vi "Source-meter - IV sweep.vi"(4 "XY Graph to update":refnum<vi>, 6 "String reference":refnum<vi>, 8 "Error In":errorcluster, 9 "Stop occurrence":refnum<k4>, 10 "IV properties":T1={"T"=0.0, "Vstart"=-0.5, "Vstop"=0.5, "Vpoints"=10.0, "Settling"=0.01, "I limit"=0.1, "Log mapping"=FALSE, "Averaging"=0.0}, 11 "Source-meter handle":T2) -> (0 "error out":errorcluster, 2 "Voltage (V)":dbl[](array[numeric]), 3 "Current (A)":dbl[](array[numeric]))   [LabVIEW 2019]
doc: "Handles I-V sweep (including data acquisition)"
uses:
  Type defs/Source-meter handle Type Def.ctl
  Type defs/Source-meter Type Def.ctl
  Custom devices/Custom source-meter settings.ctl
  Type defs/IV properties Type Def.ctl
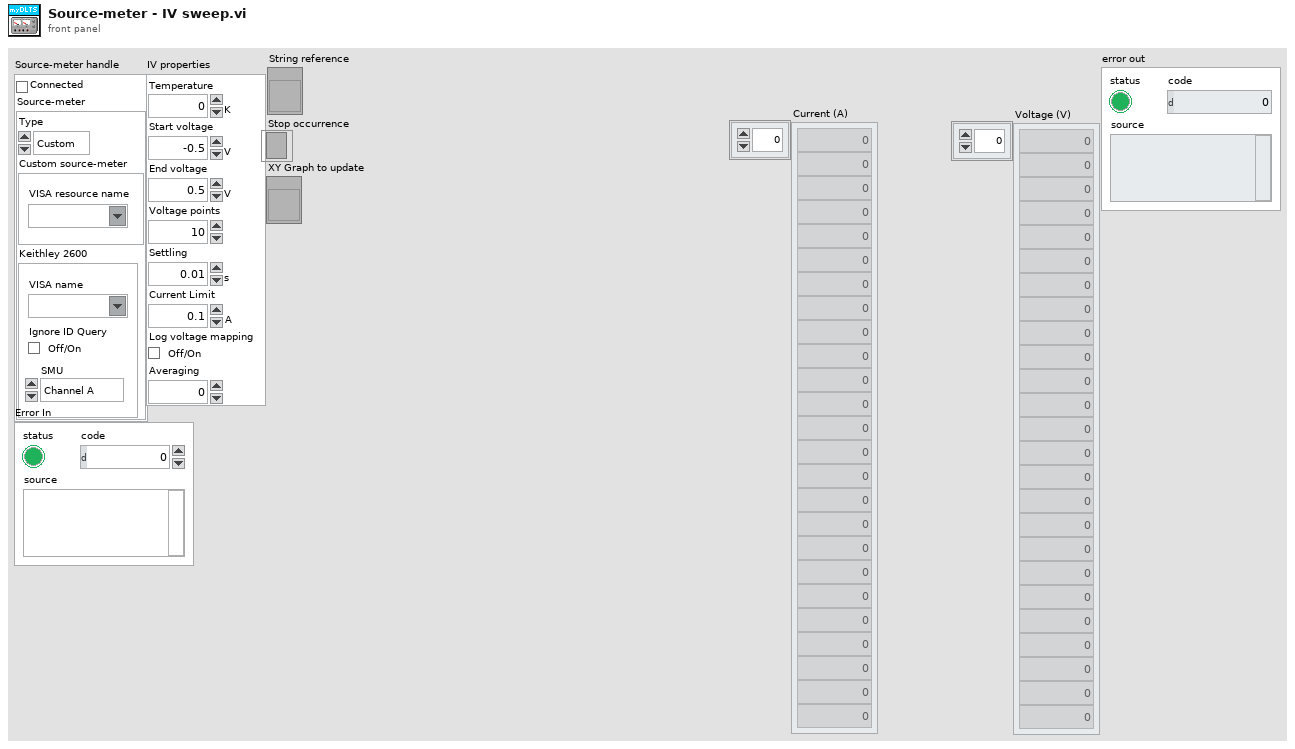
[diagram p1: front panel]
types:
  T1 = typedef "IV properties Type Def.ctl" = cluster{"T":dbl[unit], "Vstart":dbl[unit], "Vstop":dbl[unit], "Vpoints":dbl, "Settling":dbl[unit], "I limit":dbl[unit], "Log mapping":bool, "Averaging":dbl}
  T2 = typedef "Source-meter handle Type Def.ctl" = cluster{"Connected":bool, "Source-meter":T3}
  T3 = typedef "Source-meter Type Def.ctl" = cluster{"Type":enum16{"Custom", "Keithley 2600"}, "Custom source-meter":T4, "Keithley 2600":cluster{"VISA name":refnum<visa-resource-name>, "Ignore ID Query":bool, "SMU":enum16{"Channel A", "Channel B"}}}
  T4 = typedef "Custom source-meter settings.ctl" = cluster{"VISA resource name":refnum<visa-resource-name>}
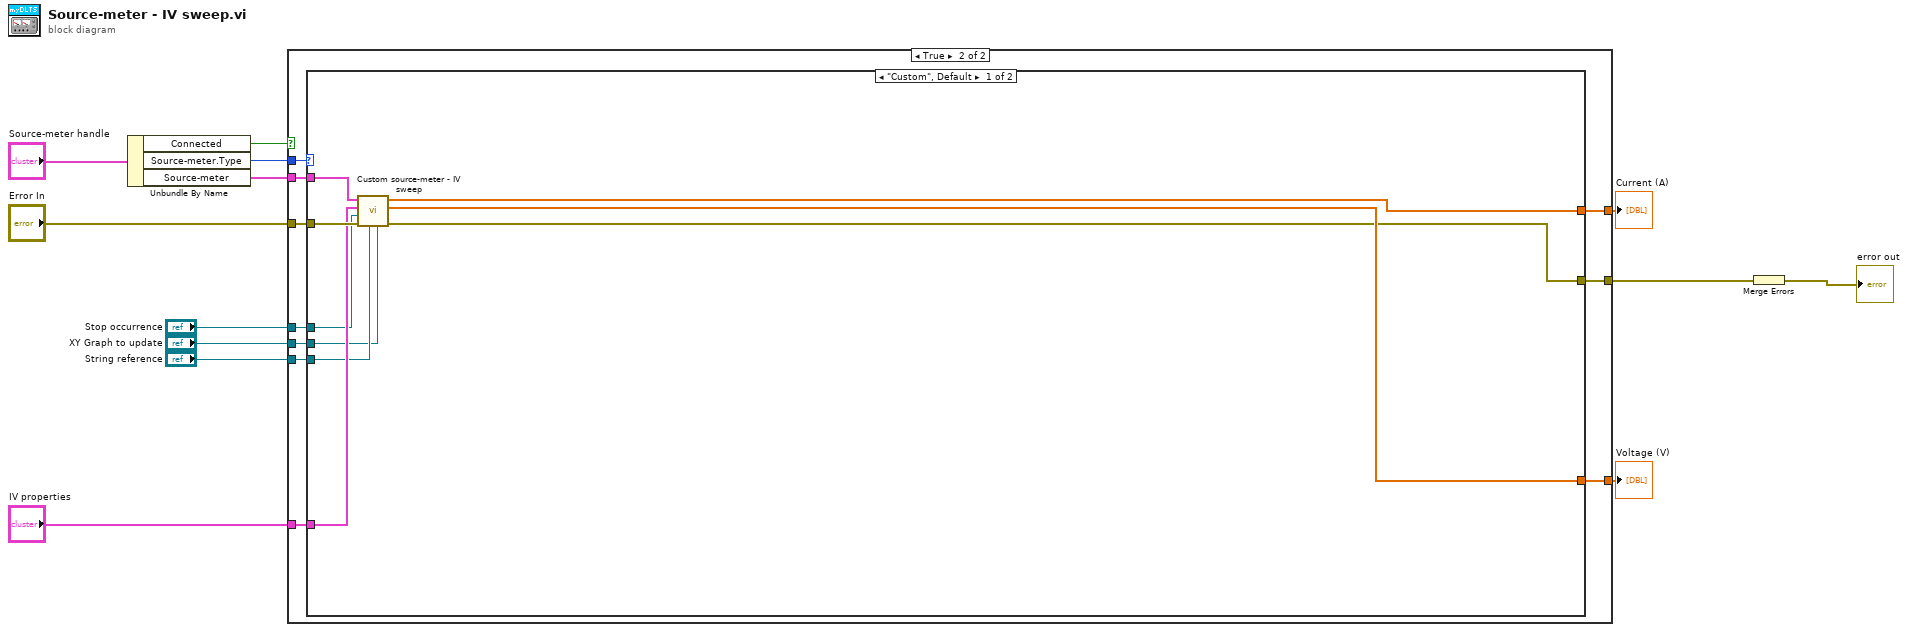
[diagram p0: block diagram]
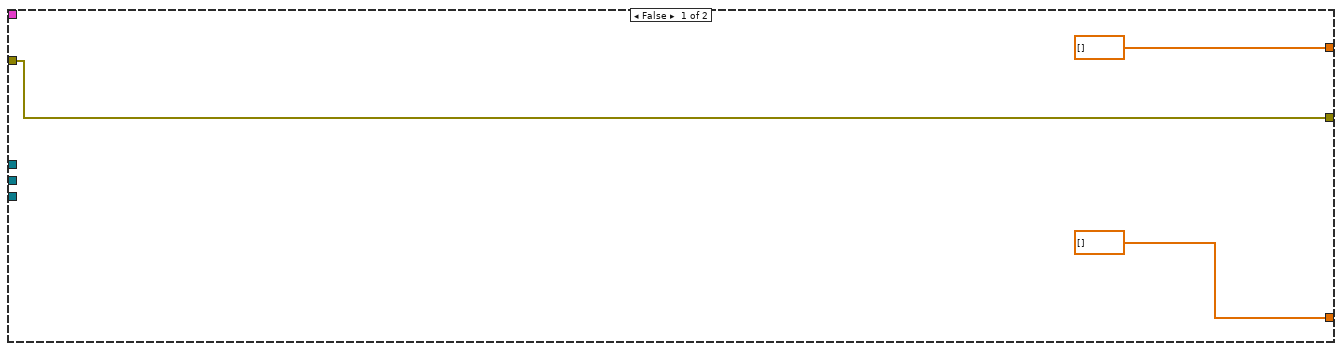
[diagram p2: hidden frame]
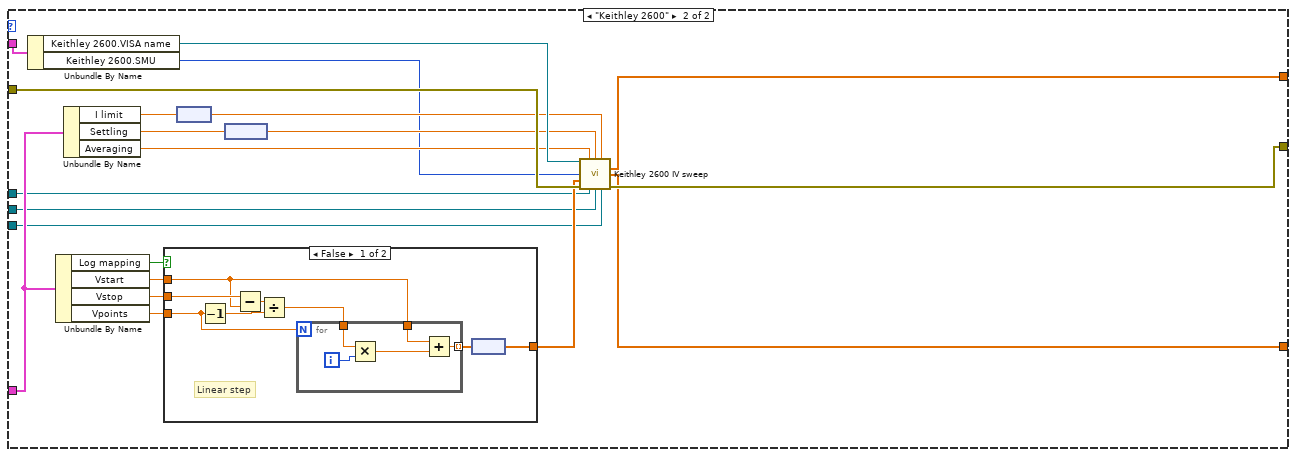
[diagram p3: hidden frame]
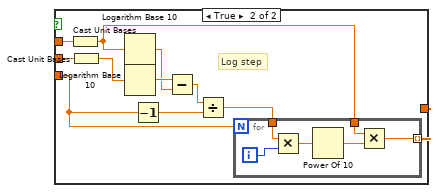
[diagram p4: hidden frame]
diagram:
  n1 = Unbundle By Name("Source-meter handle") -> ("Connected"=w12:bool, "Source-meter.Type"=w11:enum16{"Custom", "Keithley 2600"}, "Source-meter"=w10:T3)
  n2 = case shown="True" w12 {
    tunnel: w11 -> [_ w26]
    tunnel: w10 -> [_ w25]
    tunnel: "IV properties" -> [_ w24]
    tunnel: "Error In" -> [w15 w23]
    tunnel: [dbl[] [] ("Voltage (V)") w22] -> w9
    tunnel: [dbl[] [] w21] -> w8
    tunnel: [w15 w20] -> w5
    tunnel: "String reference" -> [_ w19]
    tunnel: "Stop occurrence" -> [_ w18]
    tunnel: "XY Graph to update" -> [_ w17]
    frame False {
    }
    frame True {
      n3 = case shown="\"Custom\", Default" w26 {
        tunnel: w25 -> [w34 w56]
        tunnel: w24 -> [w33 w55]
        tunnel: w23 -> [w35 w49]
        tunnel: [w31 w36] -> w22
        tunnel: [w32 w41] -> w21
        tunnel: [w30 w40] -> w20
        tunnel: w19 -> [w28 w42]
        tunnel: w18 -> [w29 w39]
        tunnel: w17 -> [w27 w38]
        frame "Custom", Default {
          n4 = call "Custom source-meter - IV sweep.vi"("XY Graph to update"=w27, "String reference"=w28, "Error In"=w35, "Stop occurrence"=w29, "IV properties"=w33, "Source-meter"=w34) -> ("Error Out"=w30:errorcluster, "Voltage (V)"=w31:dbl[], "Current (A)"=w32:dbl[])  [unwired: 3 in]
        }
        frame "Keithley 2600" {
          n5 = Unbundle By Name(w56) -> ("Keithley 2600.VISA name"=w50:refnum<visa-resource-name>, "Keithley 2600.SMU"=w37:enum16{"Channel A", "Channel B"})
          n6 = Unbundle By Name(w55) -> ("Log mapping"=w54:bool, "Vstart"=w53:dbl[unit], "Vstop"=w52:dbl[unit], "Vpoints"=w51:dbl)
          n7 = Unbundle By Name(w55) -> ("I limit"=w46:dbl[unit], "Settling"=w45:dbl[unit], "Averaging"=w43:dbl)
          n8 = case shown="False" w54 {
            tunnel: w53 -> [w59 w72]
            tunnel: w52 -> [w64 w79]
            tunnel: w51 -> [w61 w74]
            tunnel: [w57 w71] -> w48
            frame False {
              # "Linear step"
              n9 = Decrement(x=w61) -> (x-1=w62:dbl)
              n10 = Subtract(x=w64, y=w59) -> (x-y=w63:dbl[unit])
              n11 = Divide(x=w63, y=w62) -> (x/y=w60:dbl[unit])
              n12 = for {
                N: w61 -> [_]
                tunnel: w60 -> [w68]
                tunnel: w59 -> [w66]
                tunnel: [w65] -> w58 mode=indexing
                i -> [w69]
                n13 = Multiply(x=w68, y=w69) -> (x*y=w67:dbl[unit])
                n14 = Add(x=w66, y=w67) -> (x+y=w65:dbl[unit])
              }
              n15 = node(w58) -> (w57:dbl[])
            }
            frame True {
              # "Log step"
              n16 = Cast Unit Bases(0:w72) -> (2:w70:dbl)  [unwired: 1 in]
              n17 = Cast Unit Bases(0:w79) -> (2:w80:dbl)  [unwired: 1 in]
              n18 = Logarithm Base 10(1:w70) -> (0:w77:dbl)
              n19 = Logarithm Base 10(1:w80) -> (0:w78:dbl)
              n20 = Decrement(x=w74) -> (x-1=w75:dbl)
              n21 = Subtract(x=w78, y=w77) -> (x-y=w76:dbl)
              n22 = Divide(x=w76, y=w75) -> (x/y=w73:dbl)
              n23 = for {
                N: w74 -> [_]
                tunnel: w73 -> [w85]
                tunnel: w70 -> [w82]
                tunnel: [w81] -> w71 mode=indexing
                i -> [w86]
                n24 = Multiply(x=w85, y=w86) -> (x*y=w84:dbl)
                n25 = Power Of 10(x=w84) -> (10^x=w83:dbl)
                n26 = Multiply(x=w82, y=w83) -> (x*y=w81:dbl)
              }
            }
          }
          n27 = node(w46) -> (w47:dbl)
          n28 = node(w45) -> (w44:dbl)
          n29 = call "Keithley 2600 IV sweep.vi"("VISA resource name"=w50, "Filter Count (1)"=w43, "Settling (ms)"=w44, "Current limit (0.1)"=w47, "Channel (Channel A)"=w37, "Voltage points"=w48, "error in (no error)"=w49, "Stop occurrence"=w39, "XY Graph to update"=w38, "Status String Reference"=w42) -> ("Current points"=w41:dbl[], "Voltage points (Collected)"=w36:dbl[], "error out"=w40:errorcluster)  [unwired: 2 in, 1 out]
        }
      }
    }
  }
  "Current (A)" <- w8
  "Voltage (V)" <- w9
  n30 = Merge Errors(w5) -> (→"error out":errorcluster)
